vi "6UDigits.vi"() -> (0 "2D":i32[][](array[numeric]), 3 "1D":i32[](array[numeric]))   [LabVIEW 2023]
uses:
  <vilib>/numeric/Random Number (Range) U64.vi
  <vilib>/numeric/sub_Random U32.vi
panel:
  in  "Numeric":i32=3
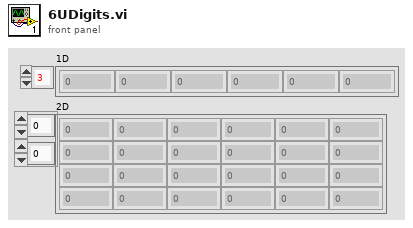
[diagram p1: front panel]
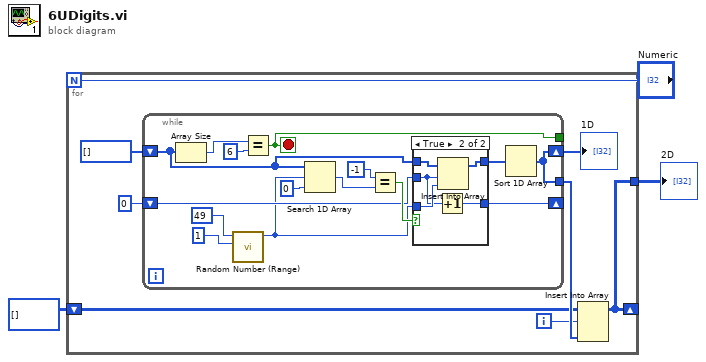
[diagram p0: block diagram]
diagram:
  n1 = for {
    N: "Numeric" -> [_]
    tunnel: [w4] -> w2
    shift-right: [w4] -> _
    shift-left: i32[][] [] -> [w5]
    i -> [w6]
    n2 = while {
      shift-right: [w11] -> w9
      shift-left: i32[] [] -> [w13]
      tunnel: [w19] -> _
      shift-right: [w16] -> _
      shift-left: u64 0 -> [w15]
      tunnel: [w11] -> w7
      stop <- w19 stop-if-true
      n3 = Array Size(array=w13) -> (size(s)=w21:i32)
      n4 = call-poly <vilib>:"Random Number (Range).vi"("lower bound (0)"=u64 1, "upper bound (100)"=u64 49) -> ("number"=w12:u64)  [unwired: 9 in]
      n5 = Equal?(x=w21, y=6) -> (x = y?=w19:bool)
      n6 = Search 1D Array(1D array=w13, element=w12, start index (0)=0 ("index")) -> (index of element=w25:i32)
      n7 = Equal?(x=-1, y=w25) -> (x = y?=w24:bool)
      n8 = case shown="True" w24 {
        tunnel: [w27 w30] -> w18
        tunnel: w13 -> [w27 w32]
        tunnel: w12 -> [_ w31]
        tunnel: [w26 w29] -> w16
        tunnel: w15 -> [w26 w28]
        frame False {
        }
        frame True {
          n9 = Increment(x=w28) -> (x+1=w29:u64)
          n10 = Insert Into Array(array=w32, index=w28, new element=w31) -> (w30:i32[])
        }
      }
      n11 = Sort 1D Array(array=w18) -> (sorted array=w11:i32[])
    }
    "1D" <- w9
    n12 = Insert Into Array(array=w5, index (row)=w6, new element=w7) -> (w4:i32[][])  [unwired: 1 in]
  }
  "2D" <- w2
